vi "BMark_MainWindow.vi"() -> ()   [LabVIEW 2013]
uses:
  controls/BMark_UI Data.ctl
  <vilib>/addons/analyzer/_analyzerctrls.llb/VIAnCtl Analysis App Info.ctl
  controls/BMark_Bookmark Data.ctl
  controls/BMark_VI_Identifier.ctl
  <vilib>/event_ctls.llb/eventvkey.ctl
  <vilib>/Utility/miscctls.llb/LVNodeAndColumnTypeDef.ctl
  <vilib>/Utility/miscctls.llb/LVRectTypeDef.ctl
  globals/BMark_User Visible Strings.vi
  support/Message Queue/BMark_Message Queue.lvlib
  support/User Event - Stop/BMark_User Event - Stop.lvlib
panel:
  in  "Scope":u16(ring) items=["Main Application Instance", "Default Bookmark Manager.lvproj"]
  in  "Search String":string
  in  "More information link":bool
  out "Warning glyph":bool
  in  "Group":enum32{"Group by Tag", "Group by VI"}(radio)
  in  "Tree":string(tree)
  in  "Help":bool
  in  "Close":bool
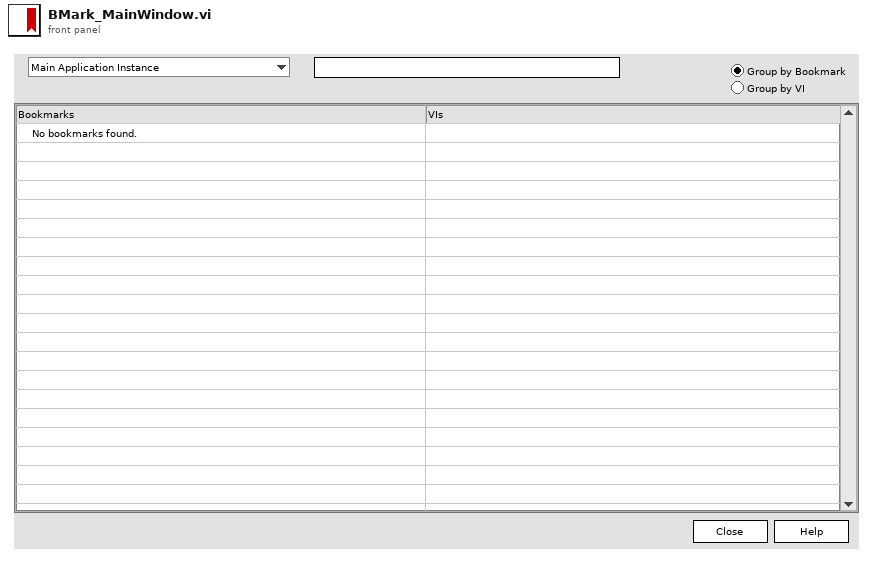
[diagram p1: front panel]
types:
  T1 = typedef "BMark_UI Data.ctl" = cluster{"Projects":refnum<vi>, "Tree":refnum<vi>, "GroupBy":refnum<vi>, "Warning glyph":refnum<vi>, "More information":refnum<vi>, "Front Panel":refnum<vi>, "GroupByVI":bool, "all projects":T2[], "bookmarks":T3[], "App Info":T2, "TopLeft Tag":string, "Collapsed Tags":string[], "Reset BM Cache?":bool, "Search String":string}
  T2 = typedef "VIAnCtl Analysis App Info.ctl" = cluster{"Project Name":string, "Target Name":string}
  T3 = typedef "BMark_Bookmark Data.ctl" = cluster{"bookmark tag":string, "full text":string, "bookmark ref":i32, "VI display name":string, "VI identifier":T4}
  T4 = typedef "BMark_VI_Identifier.ctl" = cluster{"Name":string, "Path":path, "App Info":T2}
  T5 = typedef "BMark_Message Queue.lvlib/All Message Queues.ctl" = cluster{"UI":refnum<queue>}
  T6 = typedef "eventvkey.ctl" = enum16{"ASCII", "Enter", "Return", "Shift", "Ctrl", "Alt", "Cmd", "Opt", "Caps", "NumLock", "Clear", "Break", "Up", "Down", "Left", "Right", "Insert", "Delete", "Home", "End", "PageUp", "PageDown", "Escape", "Help", "Pause", "ScrollLock", "F1", "F2", "F3", "F4", "F5", "F6", "F7", "F8", "F9", "F10", "F11", "F12", "F13", "F14", "F15", "F16", "F17", "F18", "F19", "F20", "F21", "F22", "F23", "F24", "Play", "VolumeUp", "VolumeDown", "Mute", "Two Byte Char"}
  T7 = typedef "LVRectTypeDef.ctl" = cluster{"Left":i16, "Top":i16, "Right":i16, "Bottom":i16}
  T8 = enum8{"Enabled", "Disabled", "Disabled and Grayed Out"}
  T9 = typedef "LVNodeAndColumnTypeDef.ctl" = cluster{"Node":string, "Column":i32}
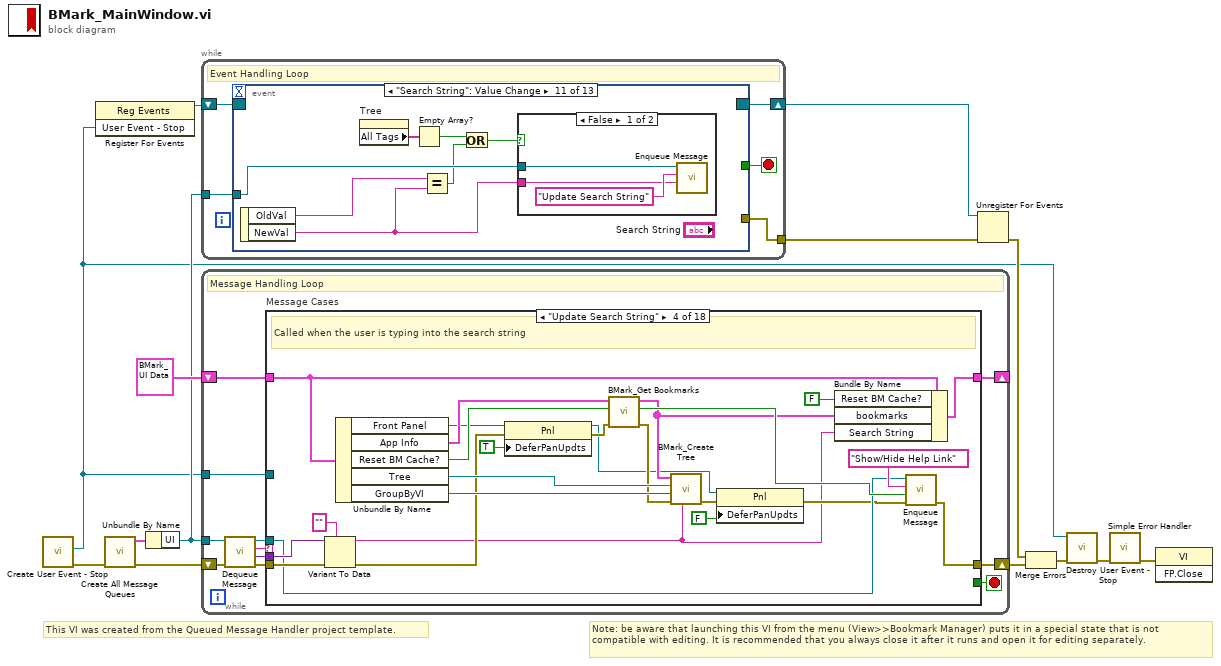
[diagram p0: block diagram]
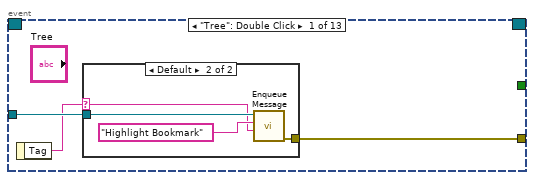
[diagram p2: hidden frame]
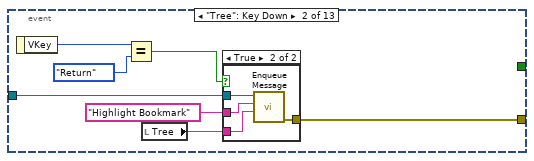
[diagram p4: hidden frame]
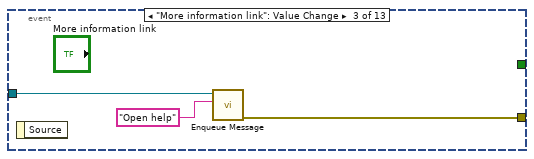
[diagram p6: hidden frame]
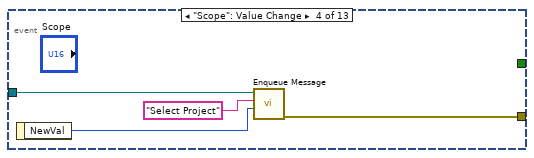
[diagram p7: hidden frame]
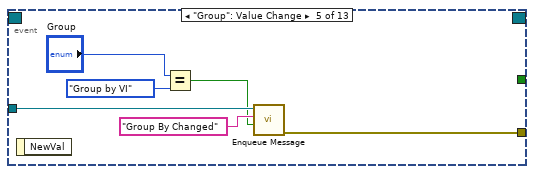
[diagram p8: hidden frame]
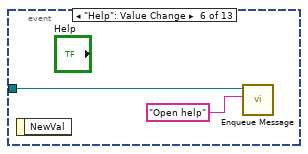
[diagram p9: hidden frame]
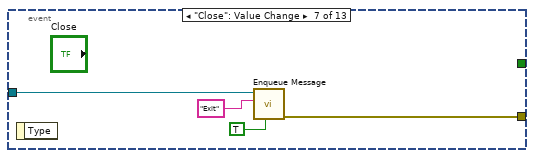
[diagram p10: hidden frame]
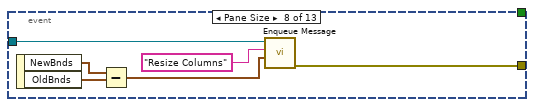
[diagram p11: hidden frame]
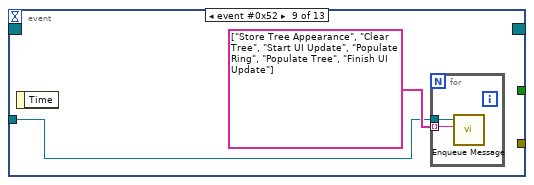
[diagram p12: hidden frame]
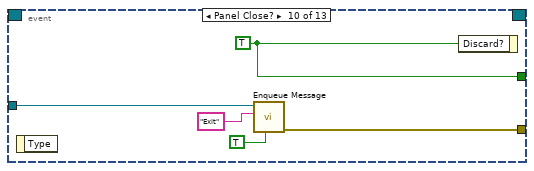
[diagram p13: hidden frame]
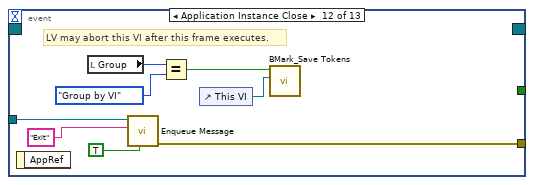
[diagram p15: hidden frame]
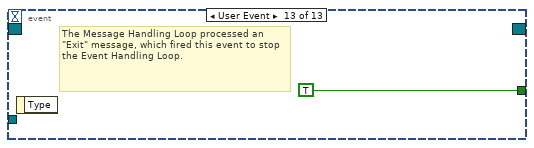
[diagram p16: hidden frame]
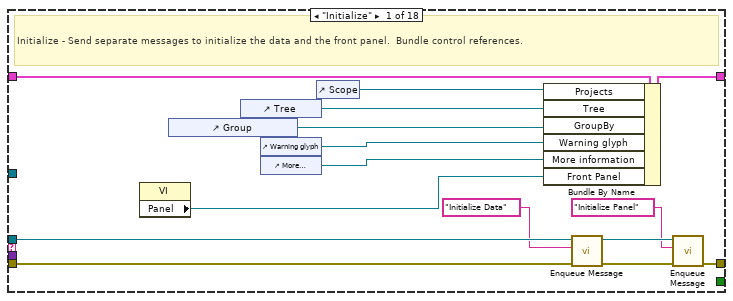
[diagram p17: hidden frame]
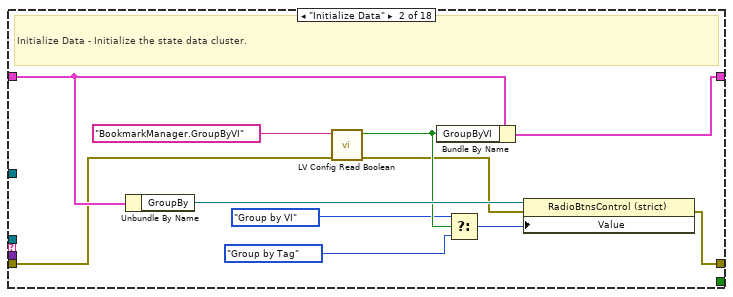
[diagram p18: hidden frame]
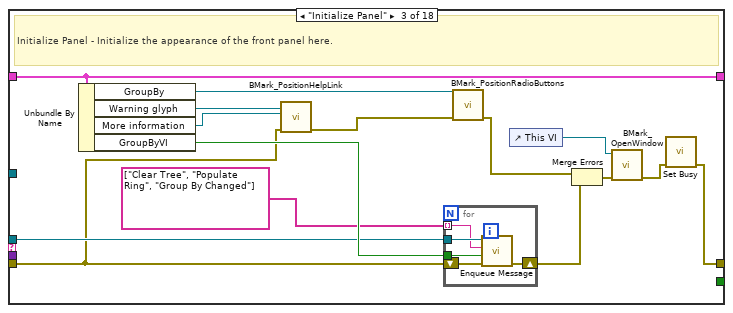
[diagram p19: hidden frame]
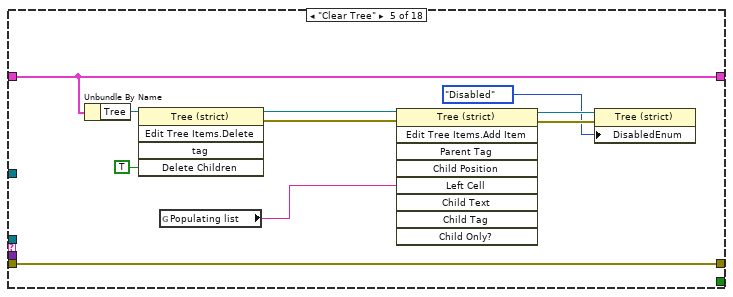
[diagram p20: hidden frame]
diagram:
  # "Note: be aware that launching this VI from the menu (View>>Bookmark Manager) puts it in a special state that is not compatible with editing. It is recommended that you always close it after it runs and open it for editing separately."
  # "This VI was created from the Queued Message Handler project template."
  n1 = call "Create User Event - Stop.vi"() -> ("error out"=w9:errorcluster, "User Event - Stop"=w1:refnum<user-event>)  [unwired: 10 in]
  n2 = register-events(w1) -> (reference out=w2:refnum<event-registration>)  [unwired: 2 in, 1 out]
  n3 = call "Create All Message Queues.vi"("error in (no error)"=w9) -> ("error out"=w5:errorcluster, "Message Queues out"=w6:T5)  [unwired: 9 in]
  n4 = Unbundle By Name(w6) -> ("UI"=w8:refnum<queue>)
  n5 = while {
    tunnel: w8 -> [w19]
    tunnel: [w18] -> w12
    shift-right: [w16] -> w13
    shift-left: w2 -> [w17]
    stop <- w15 stop-if-true
    # "Event Handling Loop"
    n6 = event shown="[10] \"Search String\": Value Change" {
      selector: w17 -> [_ _ _ _ _ _ _ _ _ _ _ _ _]
      dyn-events: [_ _ _ _ _ _ _ _ _ _ _ _ _] -> w16
      timeout: _ -> [_ _ _ _ _ _ _ _ _ _ _ _ _]
      tunnel: [_ _ _ _ _ _ _ _ _ w71 _ _ TRUE ("Discard?")] -> w15
      tunnel: w19 -> [w22 w33 w40 w44 w50 w51 w56 w61 w63 w70 w78 w89 _]
      tunnel: [w21 w32 w38 w43 w49 _ w55 w60 _ w69 _ w88 _] -> w18
      event "Tree": Double Click {
        n7 = event-data() -> ("Tag"=w20:string)  [unwired: 1 in]
        n8 = case shown="Default" w20 {
          selector: w20 -> [_ w23]
          tunnel: w22 -> [_ w26]
          tunnel: [_ w25] -> w21
          frame "" {
          }
          frame Default {
            n9 = call "Enqueue Message.vi"("Message Data"=w23, "Message"="Highlight Bookmark", "Message Queue"=w26) -> ("error out"=w25:errorcluster)  [unwired: 7 in, 1 out]
          }
        }
      }
      event "Tree": Key Down {
        n10 = event-data() -> ("VKey"=w29:T6)  [unwired: 1 in]
        n11 = Equal?(x=w29, y=eventvkey."Return") -> (x = y?=w30:bool)
        n12 = local read "Tree"() -> (w27:string)
        n13 = case shown="True" w30 {
          tunnel: w33 -> [_ w37]
          tunnel: [_ w36] -> w32
          tunnel: "Highlight Bookmark" ("Message") -> [_ w35]
          tunnel: w27 -> [_ w34]
          frame False {
          }
          frame True {
            n14 = call "Enqueue Message.vi"("Message Data"=w34, "Message"=w35, "Message Queue"=w37) -> ("error out"=w36:errorcluster)  [unwired: 7 in, 1 out]
          }
        }
      }
      event "More information link": Value Change {
        n15 = event-data() -> ()  [unwired: 1 in, 1 out]
        n16 = call "Enqueue Message.vi"("Message"="Open help", "Message Queue"=w40) -> ("error out"=w38:errorcluster)  [unwired: 8 in, 1 out]
      }
      event "Scope": Value Change {
        n17 = event-data() -> ("NewVal"=w41:u16)  [unwired: 1 in]
        n18 = call "Enqueue Message.vi"("Message Data"=w41, "Message"="Select Project", "Message Queue"=w44) -> ("error out"=w43:errorcluster)  [unwired: 7 in, 1 out]
      }
      event "Group": Value Change {
        n19 = event-data() -> ()  [unwired: 1 in, 1 out]
        n20 = Equal?(x="Group", y=enum32{"Group by Tag", "Group by VI"}."Group by VI" ("GroupBy")) -> (x = y?=w45:bool)
        n21 = call "Enqueue Message.vi"("Message Data"=w45, "Message"="Group By Changed", "Message Queue"=w50) -> ("error out"=w49:errorcluster)  [unwired: 7 in, 1 out]
      }
      event "Help": Value Change {
        n22 = event-data() -> ()  [unwired: 1 in, 1 out]
        n23 = call "Enqueue Message.vi"("Message"="Open help", "Message Queue"=w51) -> ()  [unwired: 8 in, 2 out]
      }
      event "Close": Value Change {
        n24 = event-data() -> ()  [unwired: 1 in, 1 out]
        n25 = call "Enqueue Message.vi"("Priority Message? (F)"=TRUE, "Message"="Exit", "Message Queue"=w56) -> ("error out"=w55:errorcluster)  [unwired: 7 in, 1 out]
      }
      event Pane Size {
        n26 = event-data() -> ("NewBnds"=w59:T7, "OldBnds"=w58:T7)  [unwired: 1 in]
        n27 = Subtract(x=w59, y=w58) -> (x-y=w57:T7)
        n28 = call "Enqueue Message.vi"("Message Data"=w57, "Message"="Resize Columns", "Message Queue"=w61) -> ("error out"=w60:errorcluster)  [unwired: 7 in, 1 out]
      }
      event event #0x52 {
        n29 = event-data() -> ()  [unwired: 1 in, 1 out]
        n30 = for {
          tunnel: w63 -> [w66]
          tunnel: string[] ["Store Tree Appearance", "Clear Tree", "Start UI Update", "Populate Ring", "Populate Tree", "Finish UI Update"] -> [w65] mode=indexing
          n31 = call "Enqueue Message.vi"("Message"=w65, "Message Queue"=w66) -> ()  [unwired: 8 in, 2 out]
        }
      }
      event Panel Close? {
        w71 = TRUE ("Discard?")
        n32 = event-data() -> ()  [unwired: 1 in, 1 out]
        n33 = call "Enqueue Message.vi"("Priority Message? (F)"=TRUE, "Message"="Exit", "Message Queue"=w70) -> ("error out"=w69:errorcluster)  [unwired: 7 in, 1 out]
        n34 = event-data("Discard?"=w71) -> ()  [unwired: 1 in, 1 out]
      }
      event "Search String": Value Change {
        n35 = event-data() -> ("OldVal"=w75:string, "NewVal"=w76:string)  [unwired: 1 in]
        n36 = property on="Tree" class="Tree (strict)"() -> ("All Tags"=w77:string[])  [unwired: 2 in, 2 out]
        n37 = Empty Array?(array=w77) -> (empty?=w73:bool)
        n38 = Equal?(x=w75, y=w76) -> (x = y?=w72:bool)
        n39 = Or(x=w73, y=w72) -> (x .or. y?=w74:bool)
        n40 = case shown="False" w74 {
          tunnel: w78 -> [w81 _]
          tunnel: w76 -> [w79 _]
          frame False {
            n41 = call "Enqueue Message.vi"("Message Data"=w79, "Message"="Update Search String", "Message Queue"=w81) -> ()  [unwired: 7 in, 2 out]
          }
          frame True {
          }
        }
      }
      event Application Instance Close {
        # "LV may abort this VI after this frame executes."
        n42 = event-data() -> ()  [unwired: 1 in, 1 out]
        n43 = local read "Group"() -> (w84:enum32{"Group by Tag", "Group by VI"})
        n44 = call "Enqueue Message.vi"("Priority Message? (F)"=TRUE, "Message"="Exit", "Message Queue"=w89) -> ("error out"=w88:errorcluster)  [unwired: 7 in, 1 out]
        n45 = Equal?(x=w84, y=enum32{"Group by Tag", "Group by VI"}."Group by VI" ("GroupBy")) -> (x = y?=w82:bool)
        n46 = control-ref of="This VI"() -> (w85:refnum<vi>)
        n47 = call "BMark_Save Tokens.vi"("reference"=w85, "GroupByVI"=w82) -> ()  [unwired: 10 in]
      }
      event User Event {
        # "The Message Handling Loop processed an \"Exit\" message, which fired this event to stop the Event Handling Loop."
        n48 = event-data() -> ()  [unwired: 1 in, 1 out]
      }
    }
  }
  n49 = while {
    tunnel: w8 -> [w91]
    shift-right: [w100] -> _
    shift-left: T1 {"Projects"=refnum, "Tree"=refnum, "GroupBy"=refnum, "Warning glyph"=refnum, "More information"=refnum, "Front Panel"=refnum, "GroupByVI"=FALSE, "all projects"=[], "bookmarks"=[], "App Info"={"Project Name"="", "Target Name"=""}, "TopLeft Tag"="", "Collapsed Tags"=[], "Reset BM Cache?"=FALSE, "Search String"=""} ("Data Cluster") -> [w101]
    tunnel: w1 -> [w97]
    shift-right: [w98] -> w7
    shift-left: w5 -> [w96]
    stop <- w99 stop-if-true
    # "Message Handling Loop"
    n50 = call "Dequeue Message.vi"("error in (no error)"=w96, "Message Queue"=w91) -> ("error out"=w95:errorcluster, "Message Data"=w93:variant, "Message"=w94:string, "dup Message Queue"=w92:refnum<queue>)  [unwired: 6 in]
    n51 = case "Message Cases" shown="\"Update Search String\"" w94 {
      selector: w94 -> [_ _ _ _ _ _ _ _ _ _ _ _ _ _ _ _ _ w341]
      tunnel: w92 -> [w112 _ w131 w160 _ _ w193 _ _ w228 _ _ w289 _ _ _ w336 _]
      tunnel: w95 -> [w115 w119 w130 w172 w182 w186 w196 w204 w213 w235 w236 w270 w295 w304 w312 w326 w332 _]
      tunnel: [w116 w117 w132 w159 w182 w185 w189 w204 w213 w225 w236 w264 w288 w300 w312 w325 w333 w339] -> w98
      tunnel: w101 -> [w109 w124 w142 w157 w181 w184 w190 w201 w212 w231 w250 w274 w292 w309 w311 w322 w329 w342]
      tunnel: [w108 w126 w142 w158 w181 w183 w194 w201 w211 w229 w239 w274 w291 w309 w311 w322 w329 w342] -> w100
      tunnel: [_ _ _ _ _ _ _ _ _ _ _ _ _ _ _ _ TRUE _] -> w99
      tunnel: w93 -> [_ _ _ w170 _ _ w195 _ _ _ _ w272 w294 w305 _ w324 _ _]
      tunnel: w97 -> [_ _ _ _ _ _ _ _ _ _ _ _ _ _ _ _ w331 _]
      frame "Initialize" {
        # "Initialize - Send separate messages to initialize the data and the front panel.  Bundle control references."
        n52 = property class="VI"() -> ("Panel"=w102:refnum<vi>)  [unwired: 2 in, 2 out]
        n53 = control-ref of="Group"() -> (w105:refnum<vi>)
        n54 = control-ref of="Tree"() -> (w106:refnum<vi>)
        n55 = control-ref of="Warning glyph"() -> (w104:refnum<vi>)
        n56 = control-ref of="More information link"() -> (w103:refnum<vi>)
        n57 = control-ref of="Scope"() -> (w107:refnum<vi>)
        n58 = Bundle By Name(cluster=w109, "Projects"=w107, "Tree"=w106, "GroupBy"=w105, "Warning glyph"=w104, "More information"=w103, "Front Panel"=w102) -> (w108:T1)
        n59 = call "Enqueue Message.vi"("error in (no error)"=w115, "Message"="Initialize Data", "Message Queue"=w112) -> ("error out"=w114:errorcluster, "dup Message Queue"=w113:refnum<queue>)  [unwired: 7 in]
        n60 = call "Enqueue Message.vi"("error in (no error)"=w114, "Message"="Initialize Panel", "Message Queue"=w113) -> ("error out"=w116:errorcluster)  [unwired: 7 in, 1 out]
      }
      frame "Initialize Data" {
        # "Initialize Data - Initialize the state data cluster."
        n61 = Unbundle By Name(w124) -> ("GroupBy"=w125:refnum<vi>)
        n62 = call "LV Config Read Boolean.vi"("error in"=w119, "key"="BookmarkManager.GroupByVI") -> ("error out"=w118:errorcluster, "value"=w123:bool)  [unwired: 3 in, 1 out]
        n63 = Bundle By Name(cluster=w124, "GroupByVI"=w123) -> (w126:T1)
        n64 = Select(t=enum32{"Group by Tag", "Group by VI"}."Group by VI" ("GroupBy"), s=w123, f=enum32{"Group by Tag", "Group by VI"}."Group by Tag" ("GroupBy")) -> (s? t:f=w120:enum32{"Group by Tag", "Group by VI"})
        n65 = property class="RadioBtnsControl (strict)"(reference=w125, error in=w118, "Value"=w120) -> (error out=w117:errorcluster)  [unwired: 1 out]
      }
      frame "Initialize Panel" {
        # "Initialize Panel - Initialize the appearance of the front panel here."
        n66 = Unbundle By Name(w142) -> ("GroupBy"=w141:refnum<vi>, "Warning glyph"=w139:refnum<vi>, "More information"=w138:refnum<vi>, "GroupByVI"=w140:bool)
        n67 = call "BMark_PositionHelpLink.vi"("error in (no error)"=w130, "More information"=w138, "Warning glyph"=w139) -> ("error out"=w137:errorcluster)  [unwired: 8 in]
        n68 = for {
          tunnel: w140 -> [w147]
          tunnel: w131 -> [w145]
          tunnel: string[] ["Clear Tree", "Populate Ring", "Group By Changed"] -> [w143] mode=indexing
          shift-right: [w146] -> w135
          shift-left: w130 -> [w144]
          n69 = call "Enqueue Message.vi"("error in (no error)"=w144, "Message Data"=w147, "Message"=w143, "Message Queue"=w145) -> ("error out"=w146:errorcluster)  [unwired: 6 in, 1 out]
        }
        n70 = call "BMark_PositionRadioButtons.vi"("error in (no error)"=w137, "RadioButtonsControl in"=w141) -> ("error out"=w136:errorcluster)  [unwired: 9 in]
        n71 = control-ref of="This VI"() -> (w128:refnum<vi>)
        n72 = Merge Errors(w136, w135) -> (w134:errorcluster)
        n73 = call "BMark_OpenWindow.vi"("error in (no error)"=w134, "Bookmark manager window reference"=w128) -> ("error out"=w133:errorcluster)  [unwired: 7 in, 2 out]
        n74 = call <vilib>:"Set Busy.vi"("error in (no error)"=w133) -> ("error out"=w132:errorcluster)  [unwired: 9 in, 1 out]
      }
      frame "Update Search String" {
        # "Called when the user is typing into the search string"
        n75 = Variant To Data(error in=w172, type="", Variant=w170) -> (data=w148:string, error out=w153:errorcluster)
        n76 = Unbundle By Name(w157) -> ("Front Panel"=w156:refnum<vi>, "App Info"=w168:T2, "Reset BM Cache?"=w169:bool, "Tree"=w162:refnum<vi>, "GroupByVI"=w163:bool)
        n77 = property class="Pnl"(reference=w156, error in=w153, "DeferPanUpdts"=TRUE ("Defer Panel Updates")) -> (reference out=w150:refnum<vi>, error out=w154:errorcluster)
        n78 = call "BMark_Get Bookmarks.vi"("error in (no error)"=w154, "Reset BM Cache?"=w169, "App Info"=w168) -> ("error out"=w161:errorcluster, "possible undisplayed bookmarks"=w166:bool, "bookmarks"=w164:T3[])  [unwired: 6 in]
        n79 = call "BMark_Create Tree.vi"("Search String"=w148, "error in (no error)"=w161, "GroupByVI"=w163, "TreeRef"=w162, "Bookmark info"=w164) -> ("error out"=w152:errorcluster)  [unwired: 6 in]
        n80 = property class="Pnl"(reference=w150, error in=w152, "DeferPanUpdts"=FALSE ("Defer Panel Updates")) -> (error out=w151:errorcluster)  [unwired: 1 out]
        n81 = Bundle By Name(cluster=w157, "Reset BM Cache?"=FALSE, "bookmarks"=w164, "Search String"=w148) -> (w158:T1)
        n82 = call "Enqueue Message.vi"("error in (no error)"=w151, "Message Data"=w166, "Message"="Show/Hide Help Link", "Message Queue"=w160) -> ("error out"=w159:errorcluster)  [unwired: 6 in, 1 out]
      }
      frame "Clear Tree" {
        n83 = Unbundle By Name(w181) -> ("Tree"=w180:refnum<vi>)
        n84 = invoke class="Tree (strict)" method="Edit Tree Items.Delete"(reference=w180, "Delete Children"=TRUE ("Delete Children?")) -> (reference out=w178:refnum<vi>, error out=w177:errorcluster)  [unwired: 3 in, 3 out]
        n85 = global read "BMark_User Visible Strings.vi" "Populating list"() -> (w176:string)
        n86 = invoke class="Tree (strict)" method="Edit Tree Items.Add Item"(reference=w178, error in=w177, "Left Cell"=w176) -> (reference out=w175:refnum<vi>, error out=w174:errorcluster)  [unwired: 6 in, 7 out]
        n87 = property class="Tree (strict)"(reference=w175, error in=w174, "DisabledEnum"=T8."Disabled" ("Disabled")) -> ()  [unwired: 2 out]
      }
      frame "Populate Ring" {
        # "Update the ring of all available contexts."
        n88 = call "BMark_Populate Project Ring.vi"("error in (no error)"=w186, "Data Cluster in"=w184) -> ("error out"=w185:errorcluster, "Data Cluster out"=w183:T1)  [unwired: 8 in]
      }
      frame "Group By Changed" {
        # "New Group By (VI or Bookmark) selection."
        n89 = Variant To Data(error in=w196, type=FALSE, Variant=w195) -> (data=w191:bool, error out=w187:errorcluster)
        n90 = Bundle By Name(cluster=w190, "GroupByVI"=w191) -> (w194:T1)
        n91 = for {
          tunnel: w193 -> [w200]
          tunnel: string[] ["Clear Tree", "Start UI Update", "Populate Tree", "Finish UI Update"] -> [w199] mode=indexing
          shift-right: [w198] -> w189
          shift-left: w187 -> [w197]
          n92 = call "Enqueue Message.vi"("error in (no error)"=w197, "Message"=w199, "Message Queue"=w200) -> ("error out"=w198:errorcluster)  [unwired: 7 in, 1 out]
        }
      }
      frame "Start UI Update" {
        # "Defer panel updates and turn on busy cursor."
        n93 = Unbundle By Name(w201) -> ("Front Panel"=w202:refnum<vi>)
        n94 = property class="Pnl"(reference=w202, "DeferPanUpdts"=TRUE ("Defer Panel Updates")) -> ()  [unwired: 1 in, 2 out]
        n95 = call <vilib>:"Set Busy.vi"() -> ()  [unwired: 10 in, 2 out]
      }
      frame "Store Tree Appearance" {
        # "Ignore any errors that may occur here. Being unable to store the tree appearance is not critical to the operation of the Bookmark Manager, and as such, should not generate an error that would shut down the entire UI."
        # "Store the scroll position and expanded items of the tree to restore later."
        n96 = Unbundle By Name(w212) -> ("Tree"=w208:refnum<vi>)
        n97 = property class="Tree (strict)"(reference=w208) -> (reference out=w206:refnum<vi>, "TopLeft"=w210:T9, "All Tags"=w207:string[])  [unwired: 1 in, 1 out]
        n98 = for {
          tunnel: w207 -> [w218] mode=indexing
          tunnel: w206 -> [w219]
          tunnel: [w218] -> w205 mode=indexing if=w214
          # "Item is collapsed if indent = 0 and not open"
          n99 = property class="Tree (strict)"(reference=w219, "Active Item Tag"=w218) -> ("Indent Level"=w216:i32, "Open?"=w215:bool)  [unwired: 1 in, 2 out]
          n100 = Equal To 0?(x=w216) -> (x = 0?=w217:bool)
          n101 = Compound Arithmetic op=AND(w217, invert w215) -> (w214:bool)
        }
        n102 = Unbundle By Name(w210) -> ("Node"=w209:string)
        n103 = Bundle By Name(cluster=w212, "TopLeft Tag"=w209, "Collapsed Tags"=w205) -> (w211:T1)
      }
      frame "Populate Tree" {
        # "Update the tree of bookmarks. Turn off the Reset BM Cache? flag so the cache for the current project can be used until the user changes the project ring."
        n104 = Unbundle By Name(w231) -> ("App Info"=w222:T2, "Reset BM Cache?"=w221:bool, "Tree"=w233:refnum<vi>, "GroupByVI"=w232:bool, "Search String"=w220:string)
        n105 = call "BMark_Get Bookmarks.vi"("error in (no error)"=w235, "Reset BM Cache?"=w221, "App Info"=w222) -> ("error out"=w234:errorcluster, "possible undisplayed bookmarks"=w226:bool, "bookmarks"=w230:T3[])  [unwired: 6 in]
        n106 = call "BMark_Create Tree.vi"("Search String"=w220, "error in (no error)"=w234, "GroupByVI"=w232, "TreeRef"=w233, "Bookmark info"=w230) -> ("error out"=w224:errorcluster)  [unwired: 6 in]
        n107 = Bundle By Name(cluster=w231, "Reset BM Cache?"=FALSE, "bookmarks"=w230) -> (w229:T1)
        n108 = call "Enqueue Message.vi"("error in (no error)"=w224, "Message Data"=w226, "Message"="Show/Hide Help Link", "Message Queue"=w228) -> ("error out"=w225:errorcluster)  [unwired: 6 in, 1 out]
      }
      frame "Finish UI Update" {
        # "Ignore any errors that may occur here. Being unable to restore the tree appearance is not critical to the operation of the Bookmark Manager, and as such, should not generate an error that would shut down the entire UI."
        # "Restore collapsed items (if any), restore the previous scroll position (if there is one), then undefer panel updates."
        n109 = Unbundle By Name(w250) -> ("Tree"=w241:refnum<vi>, "Collapsed Tags"=w240:string[], "TopLeft Tag"=w248:string, "Front Panel"=w249:refnum<vi>)
        n110 = case shown="Default" w248 {
          selector: w248 -> [_ w259]
          tunnel: w241 -> [w255 w258]
          tunnel: [w254 w257] -> w245
          tunnel: [w252 w259] -> w243
          tunnel: w240 -> [_ w256]
          frame "" {
            n111 = property class="Tree (strict)"(reference=w255) -> (reference out=w254:refnum<vi>, "All Tags"=w253:string[])  [unwired: 1 in, 1 out]
            n112 = Index Array(array=w253) -> (element=w252:string)  [unwired: 1 in]
          }
          frame Default {
            n113 = for {
              shift-right: [w262] -> w257
              shift-left: w258 -> [w263]
              tunnel: w256 -> [w261] mode=indexing
              n114 = property class="Tree (strict)"(reference=w263, "Active Item Tag"=w261, "Open?"=FALSE) -> (reference out=w262:refnum<vi>)  [unwired: 1 in, 1 out]
            }
          }
        }
        n115 = Bundle By Name(cluster=T9 {"Node"="", "Column"=0} ("Top Left Visible Cell"), "Node"=w243) -> (w242:T9)
        n116 = property class="Tree (strict)"(reference=w245, "TopLeft"=w242) -> (error out=w247:errorcluster)  [unwired: 1 in, 1 out]
        n117 = call <vilib>:"Clear Errors.vi"("error in (no error)"=w247) -> ("error out"=w246:errorcluster)  [unwired: 6 in]
        n118 = Bundle By Name(cluster=w250, "TopLeft Tag"="", "Collapsed Tags"=string[] []) -> (w239:T1)
        n119 = property class="Pnl"(reference=w249, error in=w246, "DeferPanUpdts"=FALSE ("Defer Panel Updates")) -> ()  [unwired: 2 out]
        n120 = call <vilib>:"Unset Busy.vi"() -> ()  [unwired: 11 in, 1 out]
      }
      frame "Highlight Bookmark" {
        # "Highlight the bookmark."
        n121 = Unbundle By Name(w274) -> ("bookmarks"=w265:T3[], "Tree"=w273:refnum<vi>)
        n122 = Variant To Data(error in=w270, type="", Variant=w272) -> (data=w266:string, error out=w269:errorcluster)
        n123 = property class="Tree (strict)"(reference=w273, error in=w269, "Active Item Tag"=w266) -> (error out=w268:errorcluster, "Indent Level"=w275:i32)  [unwired: 1 out]
        n124 = Greater Than 0?(x=w275) -> (x > 0?=w267:bool)
        n125 = case shown="True" w267 {
          tunnel: w268 -> [w276 w282]
          tunnel: [w276 w279] -> w264
          tunnel: w266 -> [_ w281]
          tunnel: w265 -> [_ w280]
          frame False {
          }
          frame True {
            n126 = call "BMark_Highlight Bookmark.vi"("error in (no error)"=w282, "bookmarks"=w280, "tag"=w281) -> ("error out"=w278:errorcluster)  [unwired: 8 in]
            n127 = call <vilib>:"Simple Error Handler.vi"("error in (no error)"=w278) -> ("error out"=w277:errorcluster)  [unwired: 4 in, 4 out]
            n128 = call <vilib>:"Clear Errors.vi"("error in (no error)"=w277) -> ("error out"=w279:errorcluster)  [unwired: 6 in]
          }
        }
      }
      frame "Select Project" {
        # "New project (or Main Application Instance) selected. Set the Reset BM Cache? flag so the Get Bookmarks VI can retrieve a fresh list of bookmarks for the newly-selected project."
        n129 = Unbundle By Name(w292) -> ("all projects"=w286:T2[])
        n130 = Variant To Data(error in=w295, type=u16 0 ("Projects"), Variant=w294) -> (data=w285:u16, error out=w290:errorcluster)
        n131 = call "BMark_Get App From Ring Selection.vi"("all projects"=w286, "Projects"=w285) -> ("App Info"=w284:T2)  [unwired: 9 in]
        n132 = Bundle By Name(cluster=w292, "Reset BM Cache?"=TRUE, "App Info"=w284) -> (w291:T1)
        n133 = for {
          tunnel: w289 -> [w298]
          shift-right: [w297] -> w288
          shift-left: w290 -> [w299]
          tunnel: string[] ["Clear Tree", "Start UI Update", "Populate Tree", "Finish UI Update"] -> [w296] mode=indexing
          n134 = call "Enqueue Message.vi"("error in (no error)"=w299, "Message"=w296, "Message Queue"=w298) -> ("error out"=w297:errorcluster)  [unwired: 7 in, 1 out]
        }
      }
      frame "Show/Hide Help Link" {
        n135 = Unbundle By Name(w309) -> ("Warning glyph"=w308:refnum<vi>, "More information"=w307:refnum<vi>)
        n136 = Variant To Data(error in=w304, type=FALSE ("Visible"), Variant=w305) -> (data=w302:bool, error out=w303:errorcluster)
        n137 = property class="Bool (strict)"(reference=w307, error in=w303, "Visible"=w302) -> (error out=w301:errorcluster)  [unwired: 1 out]
        n138 = property class="Bool (strict)"(reference=w308, error in=w301, "Visible"=w302) -> (error out=w300:errorcluster)  [unwired: 1 out]
      }
      frame "Open help" {
        n139 = call <helpdir>:"_LaunchHelp.vi"("HTML filename"="bkmk_manager_moreinfo.html") -> ()  [unwired: 6 in, 1 out]
      }
      frame "Resize Columns" {
        # "This code makes the second column of the tree \"fill\" the available space so that additional columns are never visible. Note: this doesn't work correctly if the user resizes the columns."
        n140 = Unbundle By Name(w322) -> ("Tree"=w321:refnum<vi>)
        n141 = Variant To Data(error in=w326, type=T7 {"Left"=0, "Top"=0, "Right"=0, "Bottom"=0} ("NewBnds"), Variant=w324) -> (data=w318:T7, error out=w325:errorcluster)
        n142 = Unbundle By Name(w318) -> ("Right"=w317:i16, "Left"=w316:i16)
        n143 = property class="Tree (strict)"(reference=w321, "ActiveColNum"=1 ("Active Cell:Active Column Number")) -> (reference out=w314:refnum<vi>, "Width"=w319:i32)  [unwired: 1 in, 1 out]
        n144 = Subtract(x=w317, y=w316) -> (x-y=w315:i16)
        n145 = Add(x=w319, y=w315) -> (x+y=w313:i32)
        n146 = property class="Tree (strict)"(reference=w314, "Width"=w313) -> ()  [unwired: 1 in, 2 out]
      }
      frame "Exit" {
        # "Stop the VI"
        # "Release the message queue reference"
        # "Close the Bookmark Manager window. Note that this case may not execute when quitting LabVIEW. Refer to the Application Instance Close frame in the Event Handling Loop."
        n147 = Unbundle By Name(w329) -> ("GroupByVI"=w328:bool)
        n148 = control-ref of="This VI"() -> (w327:refnum<vi>)
        n149 = call "Fire User Event - Stop.vi"("User Event - Stop"=w331) -> ("error out"=w330:errorcluster)  [unwired: 10 in]
        n150 = call "BMark_Save Tokens.vi"("reference"=w327, "GroupByVI"=w328) -> ()  [unwired: 10 in]
        n151 = Release Queue(queue=w336, error in (no error)=w332) -> (error out=w334:errorcluster)  [unwired: 1 in, 2 out]
        n152 = Merge Errors(w330, w334) -> (w333:errorcluster)
      }
      frame Default {
        # "'Default' case only runs if there is a message that isn't defined in any of the other cases.  Output a programming error."
        n153 = global read "BMark_User Visible Strings.vi" "unknown message error"() -> (w337:string)
        n154 = Format Into String(format string=w337, w341) -> (resulting string=w338:string)  [unwired: 2 in, 1 out]
        n155 = call <vilib>:"Error Cluster From Error Code.vi"("error message (\"\")"=w338, "error code (0)"=1) -> ("error out"=w339:errorcluster)  [unwired: 7 in]
      }
    }
  }
  n156 = Unregister For Events(event registration refnum=w13, error in=w12) -> (error out=w11:errorcluster)
  n157 = Merge Errors(w11, w7) -> (w10:errorcluster)
  n158 = call "Destroy User Event - Stop.vi"("error in (no error)"=w10, "User Event - Stop"=w1) -> ("error out"=w4:errorcluster)  [unwired: 9 in]
  n159 = call <vilib>:"Simple Error Handler.vi"("error in (no error)"=w4) -> ("error out"=w3:errorcluster)  [unwired: 4 in, 4 out]
  n160 = invoke class="VI" method="FP.Close"(error in=w3) -> ()  [unwired: 2 in, 3 out]
